vi "master_row.vi"() -> ()   [LabVIEW 2017]
panel:
  in  "path":string
  out "data":dynamicdata(graph)
  in  "Number of Iterations":i32
  in  "rate":dbl=100.0
  in  "number of samples":i32=100
  in  "Direction to Move":string(combo)
  in  "Pixel Size (mm)":string
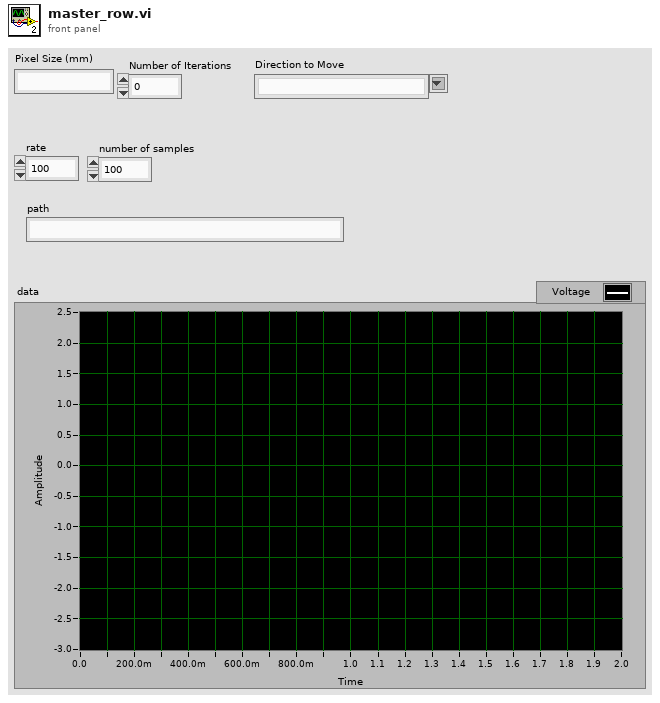
[diagram p1: front panel]
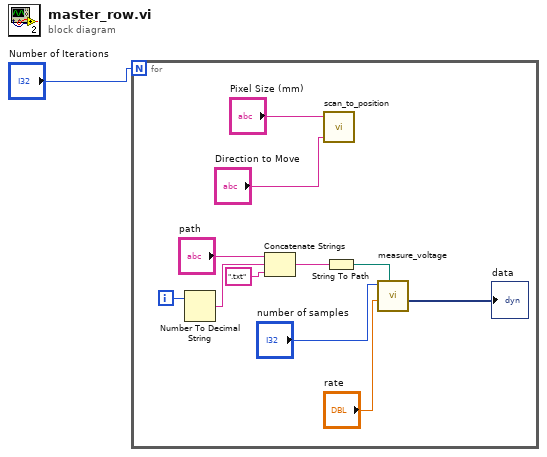
[diagram p0: block diagram]
diagram:
  n1 = for {
    N: "Number of Iterations" -> [_]
    i -> [w7]
    n2 = Number To Decimal String(number=w7) -> (decimal integer string=w6:string)  [unwired: 1 in]
    n3 = Concatenate Strings("path", w6, ".txt" ("string")) -> (w4:string)
    n4 = call "scan_to_position.vi"("Direction to Move"="Direction to Move", "Pixel Size (mm)"="Pixel Size (mm)") -> ()  [unwired: 7 in]
    n5 = String To Path(string=w4) -> (path=w3:path)
    n6 = call "measure_voltage.vi"("Filename"=w3, "rate"="rate", "number of samples"="number of samples") -> ("data"=→"data":dynamicdata)  [unwired: 8 in]
  }
